vi "Teleop.vi"(10 "Match Info":T1={"Autonomous Elapsed Seconds"=0.0, "TeleOp Elapsed Seconds"=0.0, "Disabled Elapsed Seconds"=0.0, "Visited Autonomous"=FALSE, "Visited TeleOp"=FALSE, "Visited Disabled"=FALSE, "Autonomous Settings"={"Autonomous Style"=enum."Independent", "VI Refnum"=refnum}}, 11 "Call Context":T2) -> ()   [LabVIEW 2014]
doc: "This VI is called for each TeleOp packet received from the DS where the robot is not disabled. It is often used to read from the joysticks and update I/O or to update setpoints for timed control loops. It should complete and return within 20 milliseconds or it may miss DS packets."
uses:
  <vilib>/Rock Robotics/WPI/DriverStation/WPI_DriverStationDerivedRobotMode.ctl
  <vilib>/Rock Robotics/WPI/DriverStation/WPI_DriverStationMatch Info.ctl
  <vilib>/Rock Robotics/Network Tables/SD Read Boolean.vi
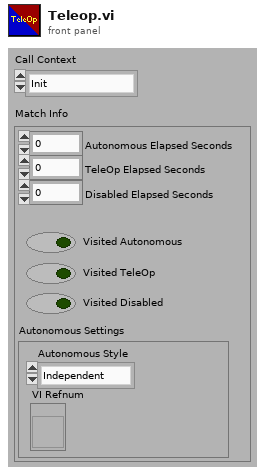
[diagram p1: front panel]
types:
  T1 = typedef "WPI_DriverStationMatch Info.ctl" = cluster{"Autonomous Elapsed Seconds":dbl, "TeleOp Elapsed Seconds":dbl, "Disabled Elapsed Seconds":dbl, "Visited Autonomous":bool, "Visited TeleOp":bool, "Visited Disabled":bool, "Autonomous Settings":cluster{"Autonomous Style":enum16{"Iterative", "Independent"}, "VI Refnum":refnum<vi>}}
  T2 = typedef "WPI_DriverStationDerivedRobotMode.ctl" = enum16{"Init", "Execute", "Stop"}
  T3 = typedef "Robot Control Outputs 2015.ctl" = cluster{"Gamepad Left Joystick left-right":dbl, "Gamepad Left Joystick up-down":dbl, "Gamepad A Button":bool, "Gamepad B Button":bool, "Gamepad X Button":bool, "Gamepad Y Button":bool, "Gamepad Left Bumper":bool, "Gamepad Right Bumper":bool, "Gamepad Back Button":bool, "Gamepad Start Button":bool, "Gamepad Left Joystick Press":bool, "Gamepad Right Joystick Press":bool, "Joystick Trigger":bool, "Joystick Thumb Button":bool, "Joystick Button 3":bool, "Joystick Button 4":bool, "Joystick Button 5":bool, "Joystick Button 6":bool, "Joystick Button 7":bool, "Joystick Button 8":bool, "Joystick Button 9":bool, "Joystick Button 10":bool, "Gamepad Left Trigger":dbl, "Gamepad Right Joystick left-right":dbl, "Gamepad Right Joystick up-down":dbl, "Joystick Left - Right":dbl, "Joystick Up-Down":dbl, "Joystick Twist":dbl, "Joystick Throttle":dbl, "Loc 1 (CB)":bool, "Loc 4 (CB)":bool, "Gamepad Right Trigger":dbl, "Loc 2 (CB)":bool, "Loc 3 (CB)":bool, "Loc 5 (CB)":bool, "Loc 6 (CB)":bool, "Loc 7 (CB)":bool, "Loc 10 (CB)":bool, "Loc 8 (CB)":bool, "Loc 9 (CB)":bool, "Loc 11 (CB)":bool, "Loc 12 (CB)":bool, "Joystick Button 11":bool, "Joystick Button 12":bool}
  T4 = typedef "Robot Commands.ctl" = cluster{"Robot Forward-Reverse":dbl, "Robot Left-Right":dbl, "Robot Twist":dbl, "Feeder Station Load Mode Enabled?":bool, "Lifter Mode (0 = Automatic Load; 1 = Manual Load; 2 = Manual Override)":dbl, "Stack Drop Command":bool, "Arm Raised?":bool, "DISABLE LIFTER":bool, "Position 1 Setpoint":bool, "Position 2 Setpoint":bool, "Position 3 Setpoint":bool, "Position 4 Setpoint":bool, "Position 5 Setpoint":bool, "Bump Lifter Down":bool, "Bump Lifter Up":bool, "Manual Load Command":bool, "Robot Centric?":bool, "Scissor Deploy/Retract":bool, "Passive Fingers":bool, "Drawbridge Raise/Lower":bool, "Twist arm up":bool, "Gyro Reset":bool, "Twist arm down":bool}
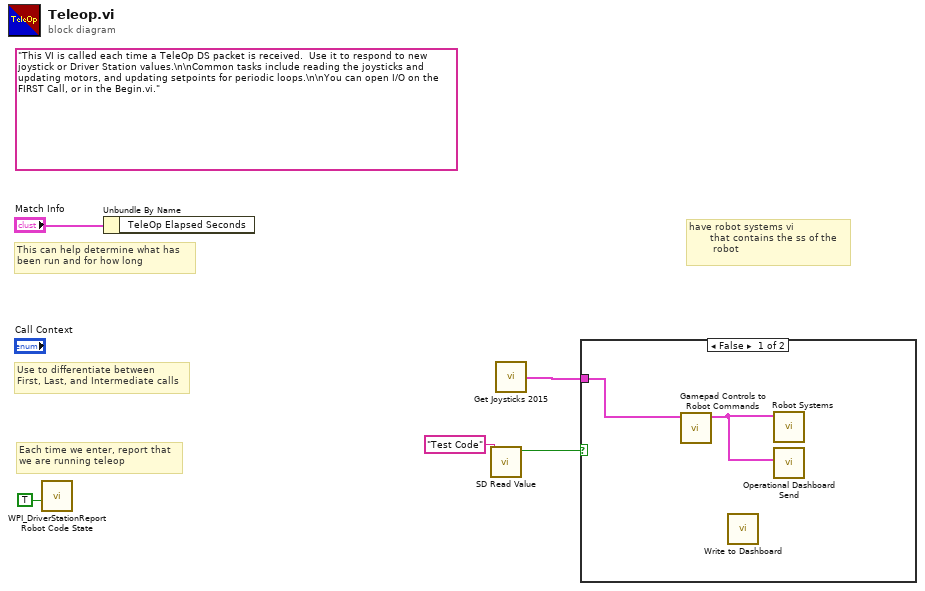
[diagram p0: block diagram]
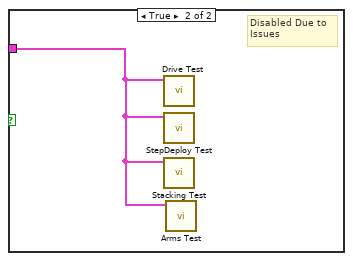
[diagram p2: hidden frame]
diagram:
  (unwired) "This VI is called each time a TeleOp DS packet is received.  Use it to respond to new joystick or Driver Station values.\n\nCommon tasks include reading the joysticks and updating motors, and updating setpoints for periodic loops.\n\nYou can open I/O on the FIRST Call, or in the Begin.vi."
  # "have robot systems vi\n       that contains the ss of the \n        robot"
  # "Each time we enter, report that\nwe are running teleop"
  # "Use to differentiate between\nFirst, Last, and Intermediate calls"
  # "This can help determine what has\nbeen run and for how long"
  n1 = call <vilib>:"WPI_DriverStationReport Robot Code State.vi"("TeleOp"=TRUE ("Autonomous")) -> ()  [unwired: 10 in, 1 out]
  n2 = Unbundle By Name("Match Info") -> ()  [unwired: 1 out]
  n3 = call-poly <vilib>:"SD Read Value.vi"("Name"="Test Code") -> ("Boolean"=w2:bool)  [unwired: 8 in, 2 out]
  n4 = call "Get Joysticks 2015.vi"() -> ("Robot Controls"=w3:T3)  [unwired: 1 in]
  n5 = case shown="False" w2 {
    tunnel: w3 -> [w7 w8]
    frame False {
      n6 = call "Gamepad Controls to Robot Commands.vi"("Robot Controls"=w7) -> ("Robot Commands"=w6:T4)  [unwired: 10 in]
      n7 = call "Write to Dashboard.vi"() -> ()  [unwired: 12 in]
      n8 = call "Robot Systems.vi"("Robot Controls"=w6) -> ()  [unwired: 11 in]
      n9 = call "Operational Dashboard Send.vi"("Robot Commands"=w6) -> ()  [unwired: 11 in]
    }
    frame True {
      # "Disabled Due to \nIssues"
      n10 = call "Drive Test.vi"("Pilot-CoPilot Gamepad Controls"=w8) -> ()  [unwired: 11 in]
      n11 = call "StepDeploy Test.vi"("Pilot-CoPilot Gamepad Controls"=w8) -> ()  [unwired: 11 in]
      n12 = call "Stacking Test.vi"("Pilot-CoPilot Gamepad Controls"=w8) -> ()  [unwired: 11 in]
      n13 = call "Arms Test.vi"("Pilot-CoPilot Gamepad Controls"=w8) -> ()  [unwired: 11 in]
    }
  }
